vi "基本波形发生器.vi"() -> ()   [LabVIEW 2012]
uses:
  <vilib>/measure/NI_MABase.lvlib
panel:
  in  "停止":bool
  in  "frequency":dbl=10.0 caption="频率" format="%0.2p"
  out "波形图":waveform(dbl)[](graph)
  in  "sampling info":cluster{"Fs":dbl, "#s":dbl}={"Fs"=1000.0, "#s"=1000.0} caption="采样信息" {"Fs" format="%.2p"}
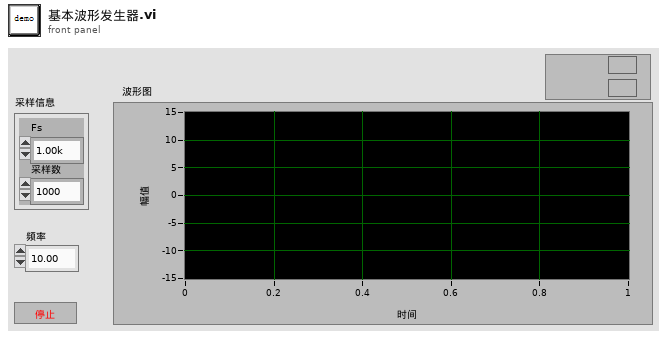
[diagram p1: front panel]
types:
  T1 = enum16{"Sine Wave", "Triangle Wave", "Square Wave", "Sawtooth Wave"}
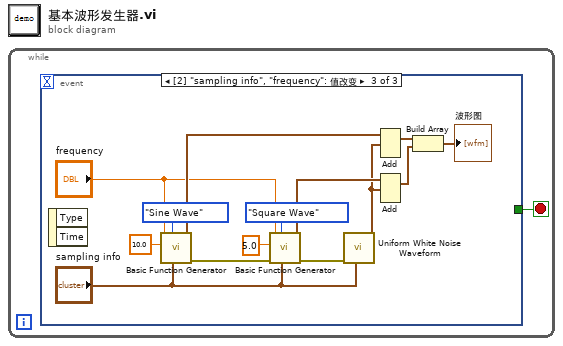
[diagram p0: block diagram]
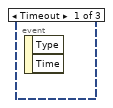
[diagram p2: hidden frame]
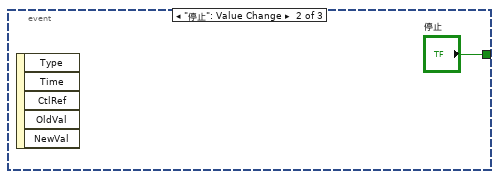
[diagram p3: hidden frame]
diagram:
  n1 = while {
    stop <- w1 stop-if-true
    n2 = event shown="[2] \"sampling info\", \"frequency\": 值改变" {
      selector: _ -> [_ _ _]
      dyn-events: _ -> [_ _ _]
      timeout: _ -> [_ _ _]
      tunnel: [_ "停止" _] -> w1
      event Timeout {
        n3 = event-data() -> ()  [unwired: 1 in, 2 out]
      }
      event "停止": Value Change {
        n4 = event-data() -> ()  [unwired: 1 in, 5 out]
      }
      event "sampling info", "frequency": Value Change {
        n5 = event-data() -> ()  [unwired: 1 in, 2 out]
        n6 = call <vilib>:"Basic Function Generator.vi"("sampling info"="sampling info", "signal type"=T1."Sine Wave", "amplitude"=10.0, "frequency"="frequency") -> ("error out"=w5:errorcluster, "signal out"=w12:waveform(dbl))  [unwired: 5 in, 1 out]
        n7 = call <vilib>:"Basic Function Generator.vi"("sampling info"="sampling info", "signal type"=T1."Square Wave", "error in (no error)"=w5, "amplitude"=5.0, "frequency"="frequency") -> ("error out"=w4:errorcluster, "signal out"=w11:waveform(dbl))  [unwired: 4 in, 1 out]
        n8 = call <vilib>:"Uniform White Noise Waveform.vi"("sampling info"="sampling info", "error in (no error)"=w4) -> ("signal out"=w10:waveform(dbl))  [unwired: 8 in, 1 out]
        n9 = Add(1:w10, 2:w12) -> (0:w9:waveform(dbl))  [unwired: 1 in, 1 out]
        n10 = Add(1:w10, 2:w11) -> (0:w8:waveform(dbl))  [unwired: 1 in, 1 out]
        n11 = Build Array(w9, w8) -> (→"波形图":waveform(dbl)[])
      }
    }
  }
